vi "FTW-DevUtil-XNode-AddItem.vi"() -> ()   [LabVIEW 2014]
panel:
  in  "Member to Add to Library":path
  in  "XNode Filepath":path
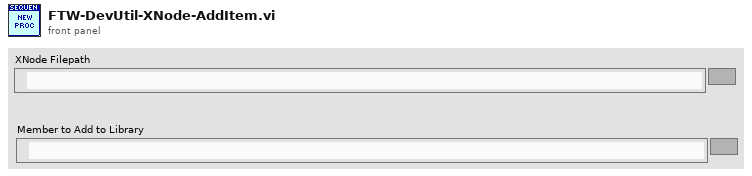
[diagram p1: front panel]
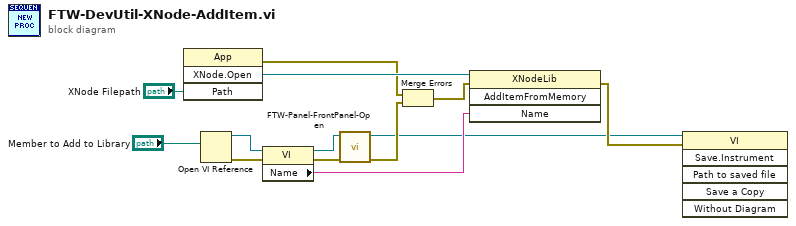
[diagram p0: block diagram]
diagram:
  n1 = invoke class="App" method="XNode.Open"("Path"="XNode Filepath") -> (error out=w7:errorcluster, "Open XNode"=w12:refnum<vi>)  [unwired: 3 in, 2 out]
  n2 = Open VI Reference(vi path="Member to Add to Library") -> (vi reference=w10:refnum<vi>, error out=w9:errorcluster)  [unwired: 5 in]
  n3 = property class="VI"(reference=w10, error in=w9) -> (reference out=w5:refnum<vi>, error out=w4:errorcluster, "Name"=w8:string)
  n4 = call "FTW-Panel-FrontPanel-Open.vi"("error in"=w4, "VI Ref"=w5) -> ("error out"=w3:errorcluster, "VI Ref out"=w1:refnum<vi>)  [unwired: 8 in]
  n5 = Merge Errors(w7, w3) -> (w6:errorcluster)
  n6 = invoke class="XNodeLib" method="AddItemFromMemory"(reference=w12, error in=w6, "Name"=w8) -> (error out=w2:errorcluster)  [unwired: 1 in, 3 out]
  n7 = invoke class="VI" method="Save.Instrument"(reference=w1, error in=w2) -> ()  [unwired: 4 in, 6 out]
